vi "Analog_Recoder.vi"(4 "External Angle In":dbl format="%#_13g", 6 "Test Name":string(combo)="DL", 7 "Lane Number":string(combo)="Lane 1", 8 "Analog Data In":dbl[](array[numeric]), 11 "Analog Array In":T1) -> (3 "Analog Array Out":T1)   [LabVIEW 2017]
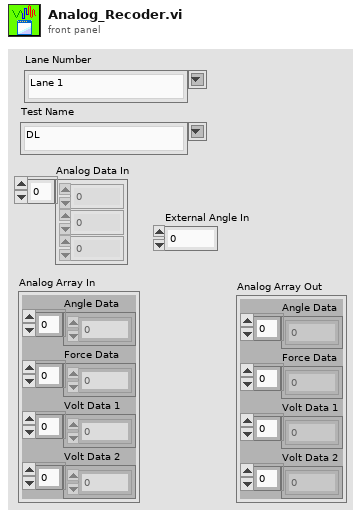
[diagram p1: front panel]
types:
  T1 = cluster{"Angle Data":dbl[], "Force Data":dbl[], "Volt Data 1":dbl[], "Volt Data 2":dbl[]}
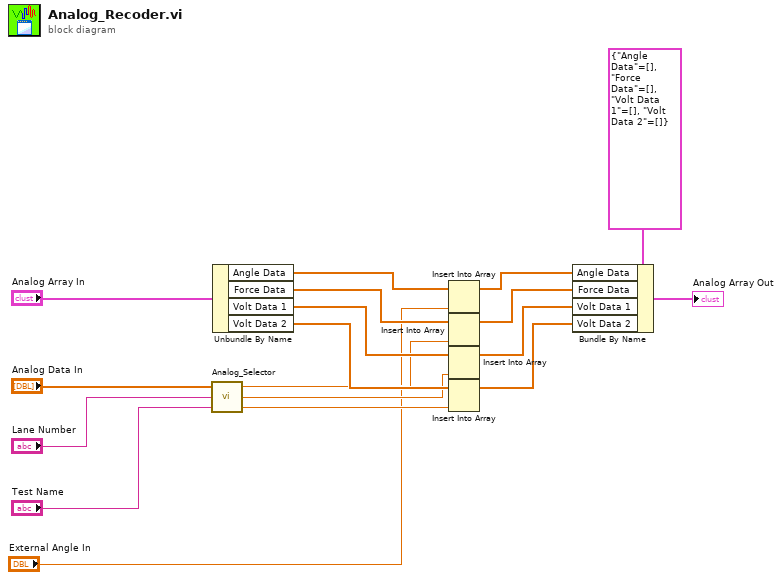
[diagram p0: block diagram]
diagram:
  n1 = call "Analog_Selector.vi"("Test Name"="Test Name", "Lane Number"="Lane Number", "Analog Data In"="Analog Data In") -> ("Volt 2"=w2:dbl, "Volt 1"=w4:dbl, "Force"=w3:dbl)
  n2 = Unbundle By Name("Analog Array In") -> ("Angle Data"=w16:dbl[], "Force Data"=w15:dbl[], "Volt Data 1"=w10:dbl[], "Volt Data 2"=w8:dbl[])
  n3 = Insert Into Array(array=w16, new element="External Angle In") -> (w18:dbl[])  [unwired: 1 in]
  n4 = Insert Into Array(array=w15, new element=w3) -> (w17:dbl[])  [unwired: 1 in]
  n5 = Insert Into Array(array=w10, new element=w4) -> (w11:dbl[])  [unwired: 1 in]
  n6 = Insert Into Array(array=w8, new element=w2) -> (w7:dbl[])  [unwired: 1 in]
  n7 = Bundle By Name(cluster=T1 {"Angle Data"=[], "Force Data"=[], "Volt Data 1"=[], "Volt Data 2"=[]} ("Analog Array Out"), "Angle Data"=w18, "Force Data"=w17, "Volt Data 1"=w11, "Volt Data 2"=w7) -> (→"Analog Array Out":T1)
